vi "Remove.vi"(8 "error in (no error)":errorcluster, 10 "Index":i32, 11 "BufferedArray in":refnum<class "BufferedArray.lvclass">) -> (0 "error out":errorcluster, 1 "Item":refnum<class>, 3 "BufferedArray out":refnum<class "BufferedArray.lvclass">)   [LabVIEW 2013, in "LapDog.Collections.v_.Lists.Implementations.lvlib" / "BufferedArray.lvclass"]
uses:
  BufferedArray.lvclass
  LapDog.Collections.Common/LapDog.Collections.v_.Common.lvlib
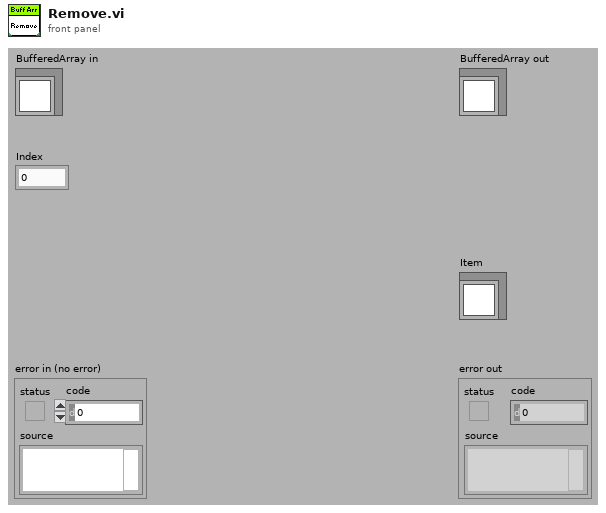
[diagram p1: front panel]
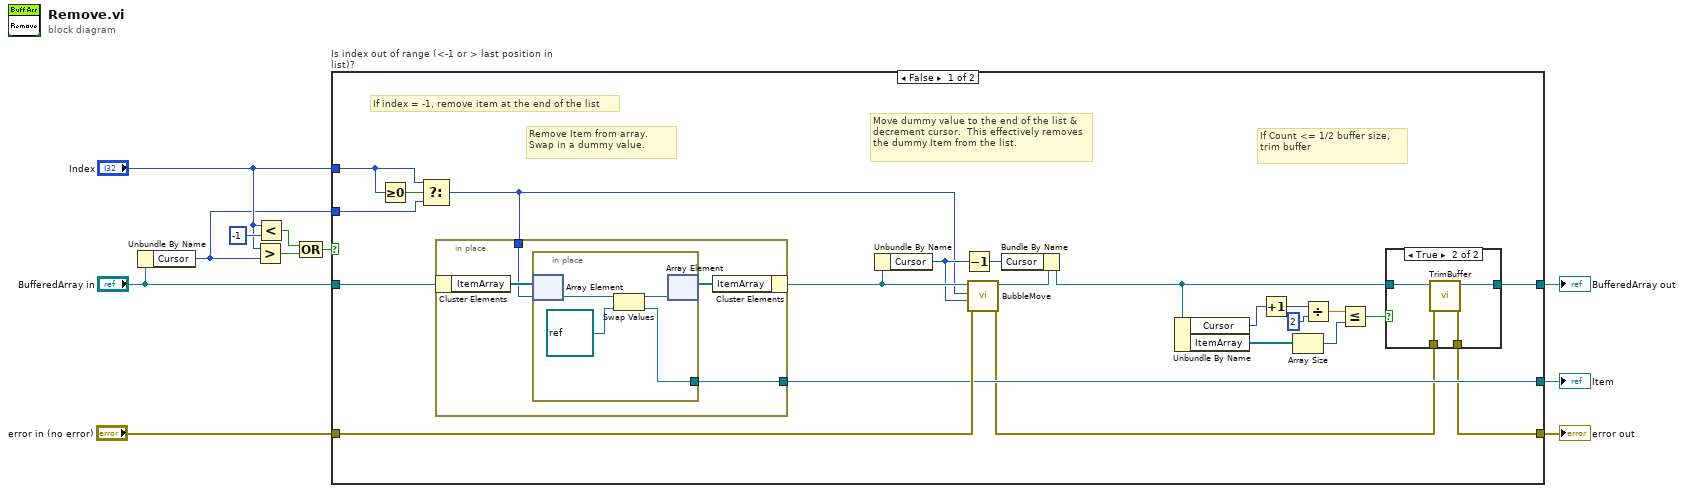
[diagram p0: block diagram]
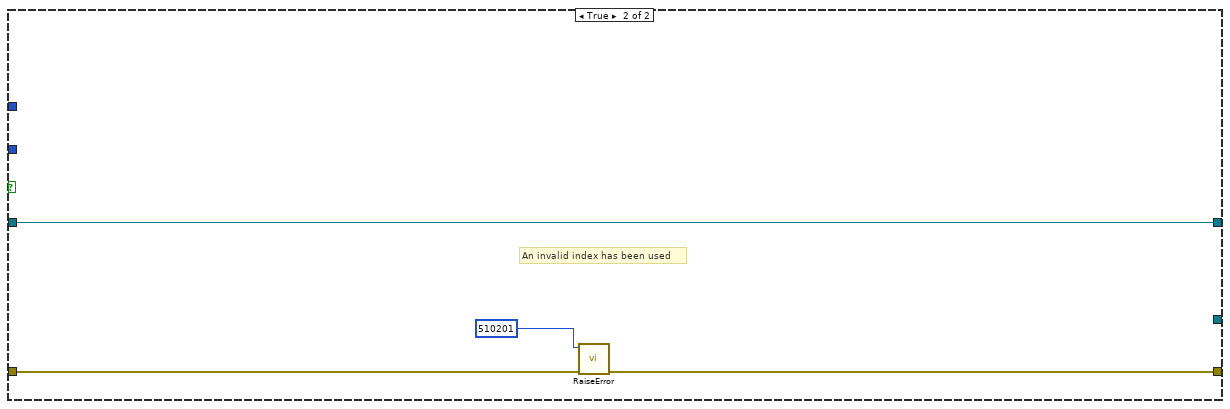
[diagram p3: hidden frame]
diagram:
  n1 = Unbundle By Name("BufferedArray in") -> ("Cursor"=w1:i32)
  n2 = Greater?(x="Index", y=w1) -> (0:w4:bool)
  n3 = Less?(x="Index", y=-1) -> (x < y?=w5:bool)
  n4 = Compound Arithmetic op=OR(w5, w4) -> (w2:bool)
  n5 = case "Is index out of range (<-1 or > last position in list)?" shown="False" w2 {
    tunnel: [w25 w51] -> w10
    tunnel: "BufferedArray in" -> [w33 w51]
    tunnel: [w22 w48] -> w8
    tunnel: "error in (no error)" -> [w31 w49]
    tunnel: "Index" -> [w14 _]
    tunnel: [w24 _] -> w7
    tunnel: w1 -> [w12 _]
    frame False {
      # "If index = -1, remove item at the end of the list"
      # "If Count <= 1/2 buffer size, trim buffer"
      # "Move dummy value to the end of the list & decrement cursor.  This effectively removes the dummy Item from the list."
      # "Remove Item from array.  Swap in a dummy value."
      n6 = Greater Or Equal To 0?(x=w14) -> (x >= 0?=w15:bool)
      n7 = Select(t=w14, s=w15, f=w12) -> (s? t:f=w13:i32)
      n8 = in-place {
        in-place-border: w13 -> [w41]
        in-place-border: [w40] -> w24
        n9 = in-place-cluster #1(w33) -> ("ItemArray"=w43:refnum<class>[])
        n10 = in-place {
          in-place-border: [w44] -> w40
          n11 = in-place-array #2(w43, w41) -> (w47:refnum<class>)
          n12 = Swap Values(12:w47, 14:refnum<class> refnum ("element")) -> (1:w45:refnum<class>, 3:w44:refnum<class>)  [unwired: 1 in]
          n13 = in-place-array #2(w45) -> (w42:refnum<class>[])  [unwired: 1 out]
        }
        n14 = in-place-cluster #1("ItemArray"=w42) -> (w30:refnum<class "BufferedArray.lvclass">)
      }
      n15 = Unbundle By Name(w30) -> ("Cursor"=w29:i32)
      n16 = Decrement(x=w29) -> (x-1=w28:i32)
      n17 = call "BubbleMove.vi"("error in (no error)"=w31, "Destination Index"=w29, "Current Index"=w13, "BufferedArray in"=w30) -> ("error out"=w23:errorcluster, "BufferedArray out"=w32:refnum<class "BufferedArray.lvclass">)  [unwired: 6 in]
      n18 = Bundle By Name(cluster=w32, "Cursor"=w28) -> (w26:refnum<class "BufferedArray.lvclass">)
      n19 = Unbundle By Name(w26) -> ("Cursor"=w21:i32, "ItemArray"=w27:refnum<class>[])
      n20 = Increment(x=w21) -> (x+1=w20:i32)
      n21 = Array Size(array=w27) -> (size(s)=w17:i32)
      n22 = Divide(x=w20, y=2) -> (x/y=w18:dbl)
      n23 = Less Or Equal?(x=w18, y=w17) -> (x <= y?=w16:bool)
      n24 = case shown="True" w16 {
        tunnel: w26 -> [w35 w39]
        tunnel: [w35 w38] -> w25
        tunnel: w23 -> [w34 w37]
        tunnel: [w34 w36] -> w22
        frame False {
        }
        frame True {
          n25 = call-dynamic "TrimBuffer.vi"("error in (no error)"=w37, "BufferedArray in"=w39) -> ("error out"=w36:errorcluster, "BufferedArray out"=w38:refnum<class "BufferedArray.lvclass">)  [unwired: 8 in]
        }
      }
    }
    frame True {
      # "An invalid index has been used"
      n26 = call "RaiseError.vi"("error in (no error)"=w49, "Error Code"=510201) -> ("error out"=w48:errorcluster)  [unwired: 9 in]
    }
  }
  "error out" <- w8
  "BufferedArray out" <- w10
  "Item" <- w7
